vi "NotifierWriter.vi"(10 "Numeric":i32) -> ()   [LabVIEW 2014]
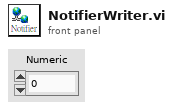
[diagram p1: front panel]
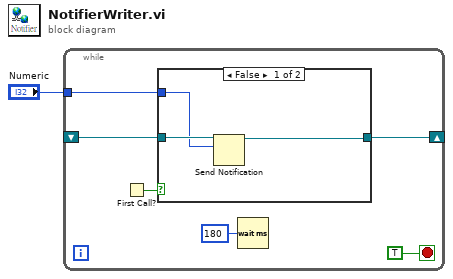
[diagram p0: block diagram]
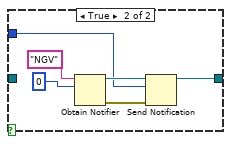
[diagram p2: hidden frame]
diagram:
  n1 = while {
    shift-right: [w5] -> _
    shift-left: _ -> [w4]
    tunnel: "Numeric" -> [w3]
    stop <- TRUE stop-if-true
    n2 = First Call?() -> (First Call?: T/F=w7:bool)
    n3 = case shown="False" w7 {
      tunnel: [w9 w12] -> w5
      tunnel: w4 -> [w10 _]
      tunnel: w3 -> [w8 w11]
      frame False {
        n4 = Send Notification(notification=w8, notifier=w10) -> (notifier out=w9:refnum<notifier>)  [unwired: 1 in, 1 out]
      }
      frame True {
        n5 = Obtain Notifier(name (unnamed)="NGV", notification data type=0 ("Numeric")) -> (notifier out=w13:refnum<notifier>, error out=w14:errorcluster)  [unwired: 2 in, 1 out]
        n6 = Send Notification(notification=w11, notifier=w13, error in (no error)=w14) -> (notifier out=w12:refnum<notifier>)  [unwired: 1 out]
      }
    }
    n7 = Wait (ms)(milliseconds to wait=u32 180) -> ()  [unwired: 1 out]
  }
